vi "slope_manual_0_20160121.vi"(0 "Reset":bool, 1 "Temp Gradient (K)":dbl, 2 "Max Temp (ºC)":dbl, 3 "Min Temp (ºC)":dbl, 4 "Temp Velocity (K/min)":dbl) -> (5 "SetPoint 1":dbl, 7 "SetPoint 2":dbl)   [LabVIEW 2011]
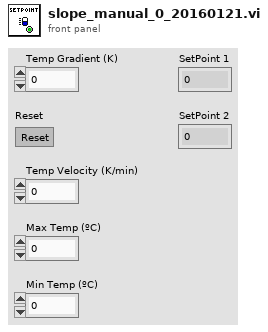
[diagram p1: front panel]
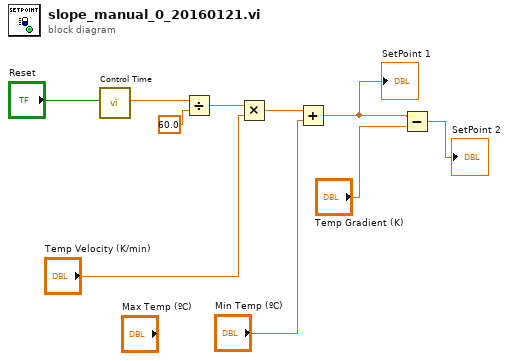
[diagram p0: block diagram]
diagram:
  n1 = call "Control Time"("Reset"="Reset") -> ("Elapsed Time (s)"=w1:dbl)  [unwired: 11 in, 7 out]
  n2 = Divide(x=w1, y=60.0) -> (x/y=w3:dbl)
  n3 = Multiply(x=w3, y="Temp Velocity (K/min)") -> (x*y=w5:dbl)
  n4 = Add(x=w5, y="Min Temp (ºC)") -> (x+y=w7:dbl)
  "SetPoint 1" <- w7
  n5 = Subtract(x=w7, y="Temp Gradient (K)") -> (x-y=→"SetPoint 2":dbl)
